vi "Get settings chain.vi"(8 "error in (no error)":errorcluster, 11 "GalvoBase in":refnum<class "InVivo_ImagingModeSPIM.lvclass">) -> (0 "error out":errorcluster, 1 "class name":string[](array[string]), 2 "settings":variant[](array[variant]), 3 "GalvoBase out":refnum<class "InVivo_ImagingModeSPIM.lvclass">)   [LabVIEW 2012, in "InVivo_ImagingModeSPIM.lvclass"]
doc: "Returns an array of variants containing the settings clusters of each class in the inheritance chain (lowest child class first), together with an array of all class names in the inheritance chain.\n\nFor classes without settings cluster, the settings chain contains empty variants."
uses:
  InVivo_ImagingModeSPIM.lvclass
  <vilib>/Distrio/Murmex/Murmex/Murmex.lvclass
  InVivo_ImagingModeSPIM.lvclass/InVivo_ImagingModeSPIM.ctl
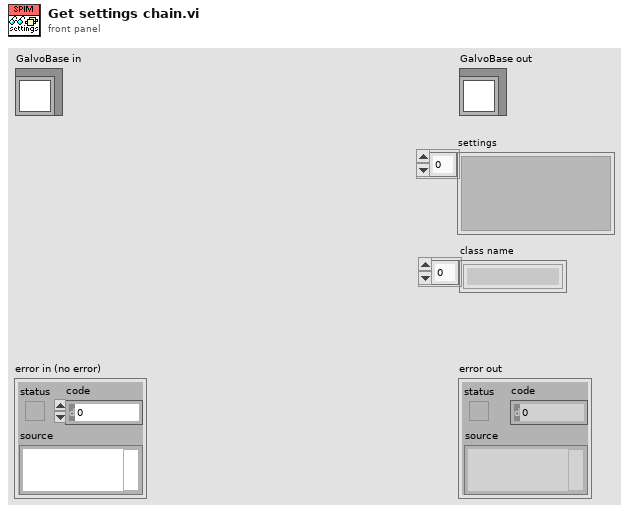
[diagram p1: front panel]
types:
  T1 = typedef "InVivo_ImagingModeSPIM.lvclass/settings_cluster.ctl" = cluster{"Frequency":dbl[unit], "Amplitude1":dbl[unit], "Phase1":dbl[unit], "DC offset1":dbl[unit], "Amplitude2":dbl[unit], "Phase2":dbl[unit], "DC offset2":dbl[unit], "Waveform type":T2, "HSYNC pulses":dbl, "pulses per pixel":i32, "digital ratio":dbl, "DC offset3":dbl[unit], "Amplitude3":dbl[unit], "Phase3":dbl[unit], "AOTFamplitude":dbl[unit], "AOTFoffset":dbl[unit], "AOTFphase":dbl[unit], "AOTFwaveform":T3, "Startaotf":bool}
  T2 = typedef "InVivo_ImagingModeSPIM.lvclass/waveform_enum.ctl" = enum16{"triangular", "sawtooth", "sinusodial"}
  T3 = typedef "InVivo_ImagingModeSPIM.lvclass/Control 4.ctl" = enum16{"Triangular", "Sawtooth", "Sinusoidal"}
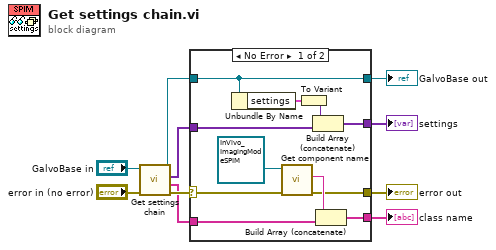
[diagram p0: block diagram]
diagram:
  n1 = call-parent "Get settings chain.vi"("error in (no error)"="error in (no error)", "MurmexBase in"="GalvoBase in") -> ("error out"=w8:errorcluster, "class name"=w7:string[], "settings"=w3:variant[], "MurmexBase out"=w4:refnum<class "InVivo_ImagingModeSPIM.lvclass">)  [unwired: 6 in]
  n2 = case shown="No Error" w8 {
    selector: w8 -> [w20 w22]
    tunnel: w7 -> [w18 w23]
    tunnel: [w17 w23] -> w6
    tunnel: [w16 w22] -> w5
    tunnel: w4 -> [w11 w25]
    tunnel: w3 -> [w15 w24]
    tunnel: [w12 w24] -> w2
    tunnel: [w11 w25] -> w1
    frame No Error {
      n3 = Unbundle By Name(w11) -> ("settings"=w14:T1)
      n4 = call <vilib>:"Get component name.vi"("error in (no error)"=w20, "Murmex in"=refnum<class "InVivo_ImagingModeSPIM.lvclass"> refnum ("Galvo.lvclass")) -> ("error out"=w16:errorcluster, "component name"=w19:string)  [unwired: 7 in, 1 out]
      n5 = To Variant(anything=w14) -> (Variant=w13:variant)
      n6 = Build Array (concatenate)(w13, w15) -> (w12:variant[])
      n7 = Build Array (concatenate)(w19, w18) -> (w17:string[])
    }
    frame Error {
    }
  }
  "error out" <- w5
  "GalvoBase out" <- w1
  "settings" <- w2
  "class name" <- w6
